vi "Get VI Metrics.vi"(8 "error in (no error)":errorcluster, 10 "VI Path":path, 11 "Code Inspector in":refnum<class "Fake Code Inspector.lvclass">) -> (0 "error out":errorcluster, 2 "VI Name":string, 3 "Code Inspector out":refnum<class "Fake Code Inspector.lvclass">, 4 "Total Diagram Count":i32, 5 "Total Node Count":i32, 6 "Uncovered Diagram Count":i32, 7 "Uncovered Node Count":i32)   [LabVIEW 2017, in "Cobertura.Tests.lvlib" / "Fake Code Inspector.lvclass"]
uses:
  Fake Code Inspector.lvclass
  Fake Code Inspector.lvclass/Fake Code Inspector.ctl
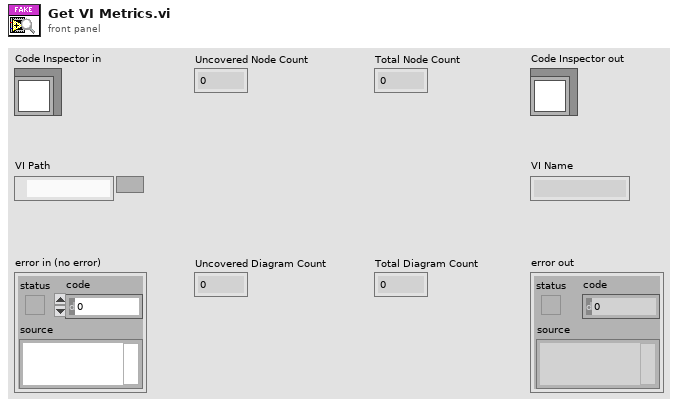
[diagram p1: front panel]
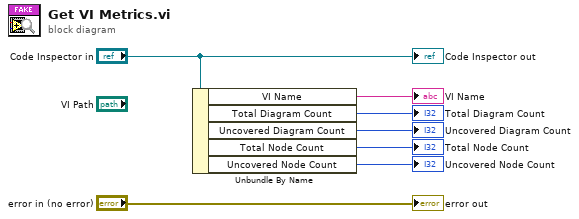
[diagram p0: block diagram]
diagram:
  n1 = Unbundle By Name("Code Inspector in") -> ("VI Name"=→"VI Name":string, "Total Diagram Count"=→"Total Diagram Count":i32, "Uncovered Diagram Count"=→"Uncovered Diagram Count":i32, "Total Node Count"=→"Total Node Count":i32, "Uncovered Node Count"=→"Uncovered Node Count":i32)
  "error out" <- "error in (no error)"
  "Code Inspector out" <- "Code Inspector in"
